vi "Terminal Test.vi"() -> ()   [LabVIEW 2020]
uses:
  Stream-Serial/Serial Client/Port Config.ctl
  Stream-Serial/Serial Client/Stop Bits.ctl
  Stream-Serial/Serial Client/Flow Control.ctl
  Stream-Serial/Serial Client/Parity.ctl
  Stream-Serial/Serial Client/Connection State.ctl
  Stream-Serial/Serial Client/Serial Client.lvclass
  C:/Program Files (x86)/National Instruments/LabVIEW 2020/vi.lib/IlluminatedG/lv-stream/Endpoint/Endpoint.lvclass
  <vilib>/IlluminatedG/lv-stream/stream/Stream.lvclass
  <vilib>/IlluminatedG/lv-stream/Endpoint/Endpoint.lvclass
panel:
  in  "Close":bool
  in  "Open":bool
  out "Log":string
  out "Connected":bool
  in  "Port Config (115200 8N1)":T1={"Baud (115200)"=115200, "Data Bits (8)"=8, "Stop Bits (1)"=10, "Flow Control"=0, "LineTerm (\\n)"="\n", "Timeout ms (10000)"=10000, "Parity (None)"=enum."None"} {"Flow Control" items=["None", "XON/XOFF", "RTS/CTS", "XON/XOFF & RTS/CTS", "DTR/DSR", "XON/XOFF & DTR/DSR"]; "Stop Bits (1)" items=["1.0"=10, "1.5"=15, "2.0"=20]}
  in  "Serial Port":refnum<visa-resource-name>
  # "Select the Port and choose the config before running the VI"
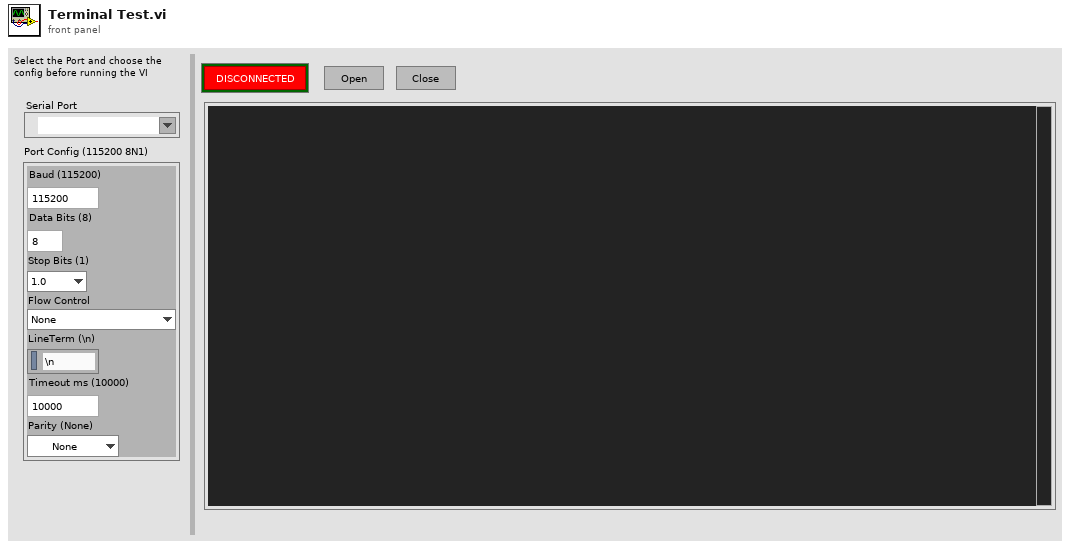
[diagram p1: front panel]
types:
  T1 = typedef "Stream-Serial.lvlib/Serial Client.lvclass/Port Config.ctl" = cluster{"Baud (115200)":u32, "Data Bits (8)":u8, "Stop Bits (1)":T2, "Flow Control":T3, "LineTerm (\\n)":string, "Timeout ms (10000)":i32, "Parity (None)":T4}
  T2 = typedef "Stream-Serial.lvlib/Serial Client.lvclass/Stop Bits.ctl" = u16
  T3 = typedef "Stream-Serial.lvlib/Serial Client.lvclass/Flow Control.ctl" = u16
  T4 = typedef "Stream-Serial.lvlib/Serial Client.lvclass/Parity.ctl" = enum16{"None", "Odd", "Even", "Mark", "Space"}
  T5 = typedef "Stream-Serial.lvlib/Serial Client.lvclass/Connection State.ctl" = enum16{"Closed", "Idle", "Connecting", "Connected", "Shutdown"}
  T6 = typedef "eventvkey.ctl" = enum16{"ASCII", "Enter", "Return", "Shift", "Ctrl", "Alt", "Cmd", "Opt", "Caps", "NumLock", "Clear", "Break", "Up", "Down", "Left", "Right", "Insert", "Delete", "Home", "End", "PageUp", "PageDown", "Escape", "Help", "Pause", "ScrollLock", "F1", "F2", "F3", "F4", "F5", "F6", "F7", "F8", "F9", "F10", "F11", "F12", "F13", "F14", "F15", "F16", "F17", "F18", "F19", "F20", "F21", "F22", "F23", "F24", "Play", "VolumeUp", "VolumeDown", "Mute", "Two Byte Char"}
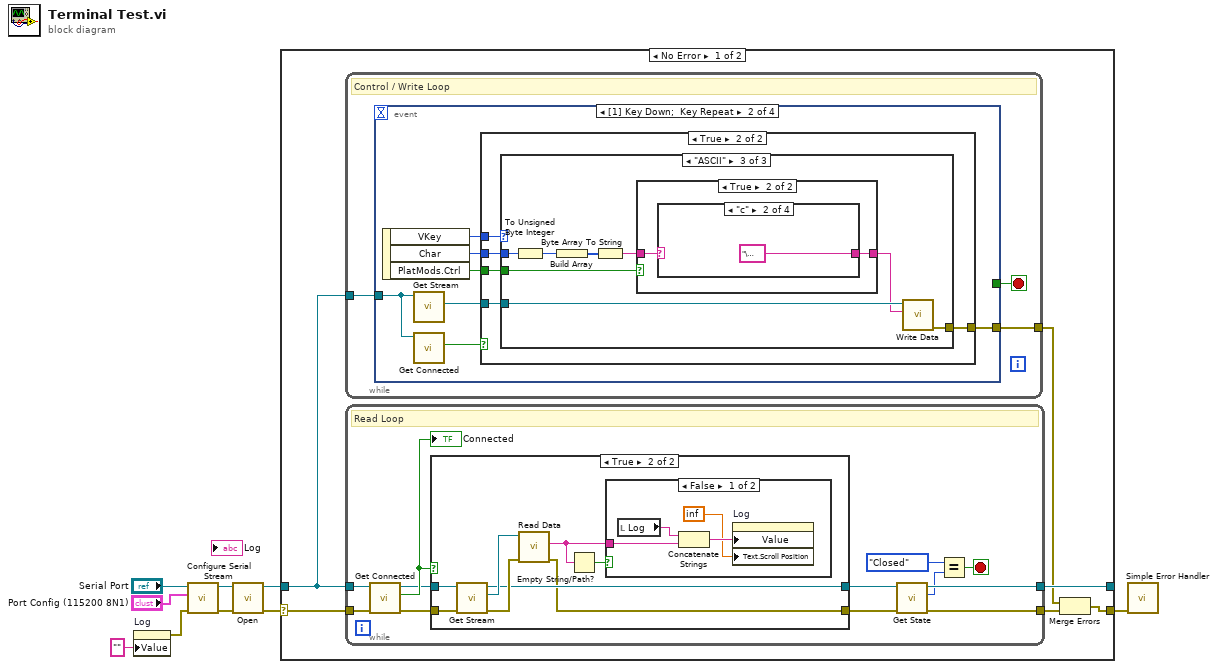
[diagram p0: block diagram]
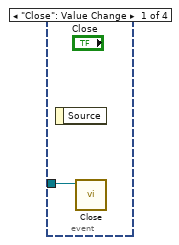
[diagram p2: hidden frame]
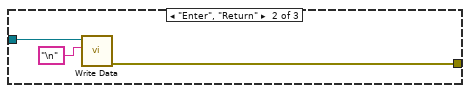
[diagram p5: hidden frame]
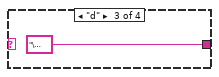
[diagram p8: hidden frame]
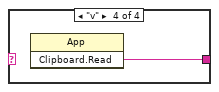
[diagram p9: hidden frame]
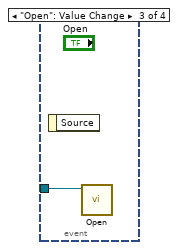
[diagram p10: hidden frame]
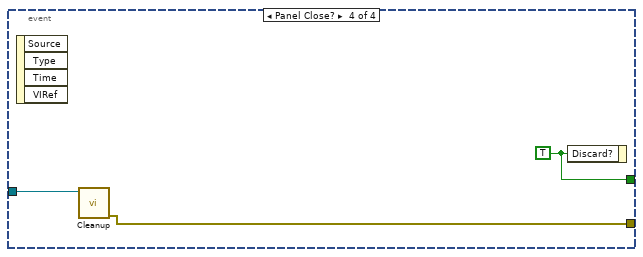
[diagram p11: hidden frame]
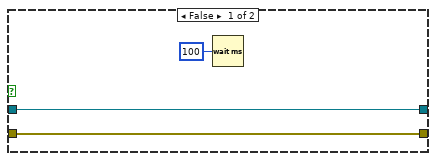
[diagram p12: hidden frame]
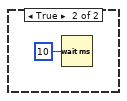
[diagram p13: hidden frame]
diagram:
  n1 = property on="Log" class="Str"("Value"="" ("Log")) -> (error out=w7:errorcluster)  [unwired: 2 in, 1 out]
  n2 = call "Configure Serial Stream.vi"("error in (no error)"=w7, "Port Config (115200 8N1)"="Port Config (115200 8N1)", "Serial Port"="Serial Port") -> ("error out"=w3:errorcluster, "Serial Client out"=w4:refnum<class "Serial Client.lvclass">)  [unwired: 7 in]
  n3 = call <vilib>:"Open.vi"("error in (no error)"=w3, "Endpoint in"=w4) -> ("error out"=w2:errorcluster, "Endpoint out"=w1:refnum<class "Serial Client.lvclass">)  [unwired: 8 in]
  n4 = case shown="No Error" w2 {
    selector: w2 -> [w15 w82]
    tunnel: w1 -> [w13 w83]
    tunnel: [w14 w83] -> _
    tunnel: [w12 w82] -> w5
    frame No Error {
      n5 = while {
        tunnel: w13 -> [w17]
        tunnel: [w16] -> w10
        stop <- w18 stop-if-true
        # "Control / Write Loop"
        n6 = event shown="[1] Key Down;  Key Repeat" {
          selector: _ -> [_ _ _ _]
          dyn-events: _ -> [_ _ _ _]
          timeout: _ -> [_ _ _ _]
          tunnel: w17 -> [w19 w21 w50 w52]
          tunnel: [_ _ _ w53] -> w18
          tunnel: [_ w23 _ w51] -> w16
          event "Close": Value Change {
            n7 = event-data() -> ()  [unwired: 1 in, 1 out]
            n8 = call <vilib>:"Close.vi"("Endpoint in"=w19) -> ()  [unwired: 9 in, 2 out]
          }
          event Key Down; Key Repeat {
            n9 = event-data() -> ("VKey"=w20:T6, "Char"=w25:i16, "PlatMods.Ctrl"=w26:bool)  [unwired: 1 in]
            n10 = call-dynamic "Get Stream.vi"("VISA Client in"=w21) -> ("Stream"=w24:refnum<class "Stream.lvclass">)  [unwired: 8 in, 2 out]
            n11 = call-dynamic "Get Connected.vi"("VISA Client in"=w21) -> ("Connected"=w22:bool)  [unwired: 8 in, 2 out]
            n12 = case shown="True" w22 {
              tunnel: w26 -> [_ w28]
              tunnel: w25 -> [_ w31]
              tunnel: w24 -> [_ w30]
              tunnel: [_ w29] -> w23
              tunnel: w20 -> [_ w27]
              frame False {
              }
              frame True {
                n13 = case shown="\"ASCII\"" w27 {
                  tunnel: w31 -> [_ _ w42]
                  tunnel: w30 -> [_ w34 w39]
                  tunnel: [_ w32 w36] -> w29
                  tunnel: w28 -> [_ _ w35]
                  frame Default {
                  }
                  frame "Enter", "Return" {
                    n14 = call-dynamic "Write Data.vi"("Data"="\n", "Stream in"=w34) -> ("error out"=w32:errorcluster)  [unwired: 8 in, 1 out]
                  }
                  frame "ASCII" {
                    n15 = To Unsigned Byte Integer(number=w42) -> (unsigned 8bit integer=w41:u8)
                    n16 = Build Array(w41) -> (w40:u8[])
                    n17 = Byte Array To String(unsigned byte array=w40) -> (string=w38:string)
                    n18 = case shown="True" w35 {
                      tunnel: w38 -> [w43 w45]
                      tunnel: [w43 w44] -> w37
                      frame False {
                      }
                      frame True {
                        n19 = case shown="\"c\"" w45 {
                          selector: w45 -> [w46 _ _ _]
                          tunnel: [w46 "\u0003" ("Data") "\u0004" ("Data") w49] -> w44
                          frame Default {
                          }
                          frame "c" {
                          }
                          frame "d" {
                          }
                          frame "v" {
                            n20 = invoke class="App" method="Clipboard.Read"() -> ("Read Clipbrd"=w49:string)  [unwired: 3 in, 2 out]
                          }
                        }
                      }
                    }
                    n21 = call-dynamic "Write Data.vi"("Data"=w37, "Stream in"=w39) -> ("error out"=w36:errorcluster)  [unwired: 8 in, 1 out]
                  }
                }
              }
            }
          }
          event "Open": Value Change {
            n22 = event-data() -> ()  [unwired: 1 in, 1 out]
            n23 = call <vilib>:"Open.vi"("Endpoint in"=w50) -> ()  [unwired: 9 in, 2 out]
          }
          event Panel Close? {
            w53 = TRUE ("Discard?")
            n24 = event-data() -> ()  [unwired: 1 in, 4 out]
            n25 = call-dynamic "Cleanup.vi"("VISA Client in"=w52) -> ("error out"=w51:errorcluster)  [unwired: 10 in]
            n26 = event-data("Discard?"=w53) -> ()  [unwired: 1 in, 1 out]
          }
        }
      }
      n27 = while {
        tunnel: w13 -> [w65]
        tunnel: w15 -> [w64]
        tunnel: [w58] -> w14
        tunnel: [w57] -> w11
        stop <- w54 stop-if-true
        # "Read Loop"
        n28 = call-dynamic "Get Connected.vi"("error in (no error)"=w64, "VISA Client in"=w65) -> ("error out"=w63:errorcluster, "Connected"=w62:bool, "VISA Client out"=w61:refnum<class "Serial Client.lvclass">)  [unwired: 7 in]
        "Connected" <- w62
        n29 = case shown="True" w62 {
          tunnel: w61 -> [w68 w76]
          tunnel: w63 -> [w67 w75]
          tunnel: [w68 w70] -> w60
          tunnel: [w67 w69] -> w59
          frame False {
            n30 = Wait (ms)(milliseconds to wait=u32 100) -> ()  [unwired: 1 out]
          }
          frame True {
            n31 = call-dynamic "Get Stream.vi"("error in (no error)"=w75, "VISA Client in"=w76) -> ("error out"=w73:errorcluster, "Stream"=w74:refnum<class "Stream.lvclass">, "VISA Client out"=w70:refnum<class "Serial Client.lvclass">)  [unwired: 7 in]
            n32 = call-dynamic "Read Data.vi"("error in (no error)"=w73, "Stream in"=w74) -> ("error out"=w69:errorcluster, "Data"=w72:string)  [unwired: 7 in, 1 out]
            n33 = Empty String/Path?(string/path=w72) -> (empty?=w71:bool)
            n34 = case shown="False" w71 {
              tunnel: w72 -> [w77 _]
              frame False {
                n35 = local read "Log"() -> (w80:string)
                n36 = Concatenate Strings(w80, w77) -> (w79:string)
                n37 = property on="Log" class="Str"("Value"=w79, "Text.Scroll Position"=inf) -> ()  [unwired: 2 in, 2 out]
              }
              frame True {
                n38 = Wait (ms)(milliseconds to wait=u32 10) -> ()  [unwired: 1 out]
              }
            }
          }
        }
        n39 = call "Get State.vi"("error in (no error)"=w59, "VISA Client in"=w60) -> ("error out"=w57:errorcluster, "State"=w56:T5, "VISA Client out"=w58:refnum<class "Serial Client.lvclass">)  [unwired: 7 in]
        n40 = Equal?(x=Connection_State."Closed", y=w56) -> (x = y?=w54:bool)
      }
      n41 = Merge Errors(w10, w11) -> (w12:errorcluster)
    }
    frame Error {
    }
  }
  n42 = call <vilib>:"Simple Error Handler.vi"("error in (no error)"=w5) -> ()  [unwired: 4 in, 5 out]
